vi "WLAN - TV - RW - UTIL - TestVectors_11B.vi"(0 "TV_IQComposite_11B":T2={"Standard"=0, "DSSS Demod Parameters"={"DSSS Auto Compute Acquisition Length Enabled"=0, "DSSS Equalization Enabled"=0, "DSSS Header Detection Enabled"=0, "DSSS MAC FCS Check Enabled"=0, "DSSS Measurement Start Location"=0, "DSSS Phase Tracking Method"=0, "DSSS Maximum Chips Used"=0, "DSSS Reference Pulse Shaping Filter"=0, "DSSS Reference Pulse Shaping Filter Coefficient"=0.0, "# Avg"=1024, "# Iterations"=1024, "DSSS Power Ramp Enabled"=0}, "DSSS Gen Paramaters"=[], "Measurement Enabled ? "=FALSE} {"DSSS Gen Paramaters"."Center Frequency(Hz)" format="%#_6p"; "DSSS Gen Paramaters"."Generation Properties"."DSSS Data Rate (Mbps)" items=["1", "2", "5.5 CCK", "5.5 PBCC", "11 CCK", "11 PBCC", "22", "33"]; "DSSS Demod Parameters"."DSSS Power Ramp Enabled" items=["False", "True"]; "DSSS Demod Parameters"."DSSS Auto Compute Acquisition Length Enabled" items=["False", "True"]; "DSSS Demod Parameters"."DSSS Phase Tracking Method" items=["Standard", "Instantaneous"]; "DSSS Demod Parameters"."DSSS Equalization Enabled" items=["False", "True"]; "DSSS Demod Parameters"."DSSS Reference Pulse Shaping Filter" items=["Rectangular", "Raised Cosine", "Root Raised Cosine", "Gaussian"]; "DSSS Demod Parameters"."DSSS MAC FCS Check Enabled" items=["False", "True"]; "DSSS Demod Parameters"."DSSS Header Detection Enabled" items=["False", "True"]; "Standard" items=["80211A/G/J/P OFDM", "80211B/G DSSS", "80211G DSSSOFDM", "80211N MIMOOFDM", "80211AC MIMOOFDM"]}, 1 "11b_Meas_Config":path, 3 "TV_802_11b":path, 9 "TV Paramaters":T1) -> ()   [LabVIEW 2011]
uses:
  Includes/WLAN - TV - RW - INC - TV_IQComposite_11B.ctl
  Includes/WLAN - TV - RW - INC - TV_DSSS Demod.ctl
  Includes/WLAN - TV - RW - INC - TV_Parameters.ctl
  Includes/WLAN - TV - RW - INC - Tx_Meas_Settings_DSSS_String.ctl
  <vilib>/Utility/file.llb/Write To Spreadsheet File (string).vi
panel:
  in  "Measurement Type 802.11G":enum32{"Tx Measurement", "Tx Measurement 2"}(tab)
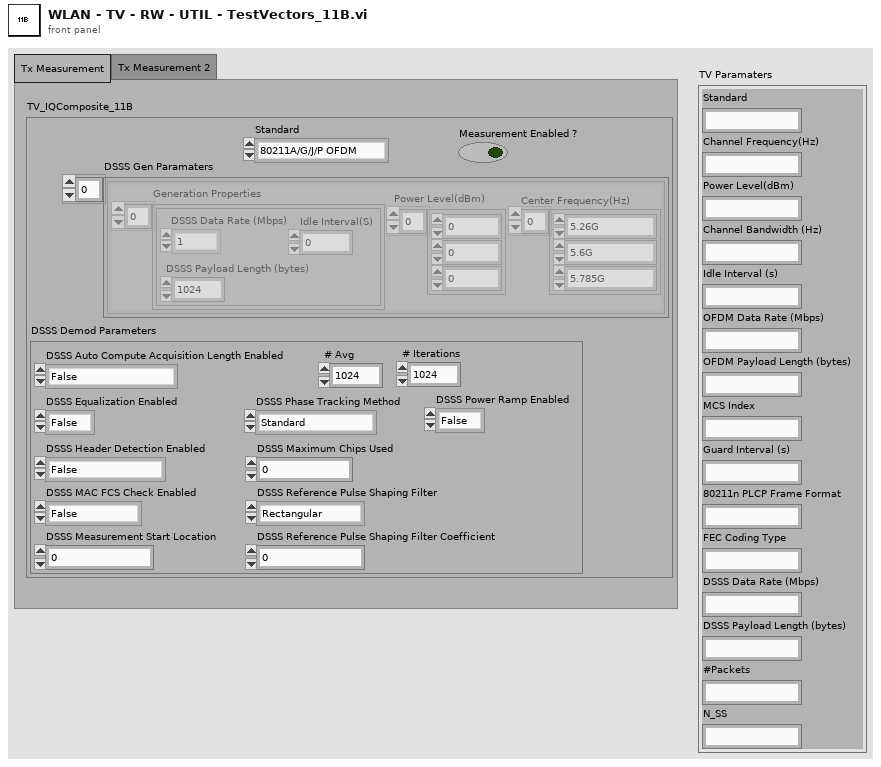
[diagram p1: front panel]
types:
  T1 = typedef "WLAN - TV - RW - INC - TV_Parameters.ctl" = cluster{"Standard ":string, "Channel Frequency(Hz)":string, "Power Level(dBm)":string, "Channel Bandwidth (Hz)":string, "Idle Interval (s)":string, "OFDM Data Rate (Mbps)":string, "OFDM Payload Length (bytes)":string, "MCS Index":string, "Guard Interval (s)":string, "80211n PLCP Frame Format":string, "FEC Coding Type":string, "DSSS Data Rate (Mbps)":string, "DSSS Payload Length (bytes)":string, "#Packets":string, "N_SS":string}
  T2 = typedef "WLAN - TV - RW - INC - TV_IQComposite_11B.ctl" = cluster{"Standard":i32, "DSSS Demod Parameters":T3, "DSSS Gen Paramaters":cluster{"Generation Properties":cluster{"DSSS Data Rate (Mbps)":i32, "DSSS Payload Length (bytes)":i32, "Idle Interval(S)":dbl}[], "Power Level(dBm)":dbl[], "Center Frequency(Hz)":dbl[]}[], "Measurement Enabled ? ":bool}
  T3 = typedef "WLAN - TV - RW - INC - TV_DSSS Demod.ctl" = cluster{"DSSS Auto Compute Acquisition Length Enabled":i32, "DSSS Equalization Enabled":i32, "DSSS Header Detection Enabled":i32, "DSSS MAC FCS Check Enabled":i32, "DSSS Measurement Start Location":i32, "DSSS Phase Tracking Method":i32, "DSSS Maximum Chips Used":i32, "DSSS Reference Pulse Shaping Filter":i32, "DSSS Reference Pulse Shaping Filter Coefficient":dbl, "# Avg":i32, "# Iterations":i32, "DSSS Power Ramp Enabled":i32}
  T4 = typedef "WLAN - TV - RW - INC - Tx_Meas_Settings_DSSS_String.ctl" = cluster{"DSSS Auto Compute Acquisition Length Enabled":string, "DSSS Equalization Enabled":string, "DSSS Header Detection Enabled":string, "DSSS MAC FCS Check Enabled":string, "DSSS Measurement Start Location":string, "DSSS Phase Tracking Method":string, "DSSS Maximum Chips Used":string, "DSSS Reference Pulse Shaping Filter":string, "DSSS Reference Pulse Shaping Filter Coefficient":string, "#Avg":string, "#Iterations":string, "DSSS Ramp Enabled ":string}
  T5 = cluster{"Generation Properties":cluster{"DSSS Data Rate (Mbps)":i32, "DSSS Payload Length (bytes)":i32, "Idle Interval(S)":dbl}[], "Power Level(dBm)":dbl[], "Center Frequency(Hz)":dbl[]}[]
  T6 = cluster{"DSSS Data Rate (Mbps)":i32, "DSSS Payload Length (bytes)":i32, "Idle Interval(S)":dbl}[]
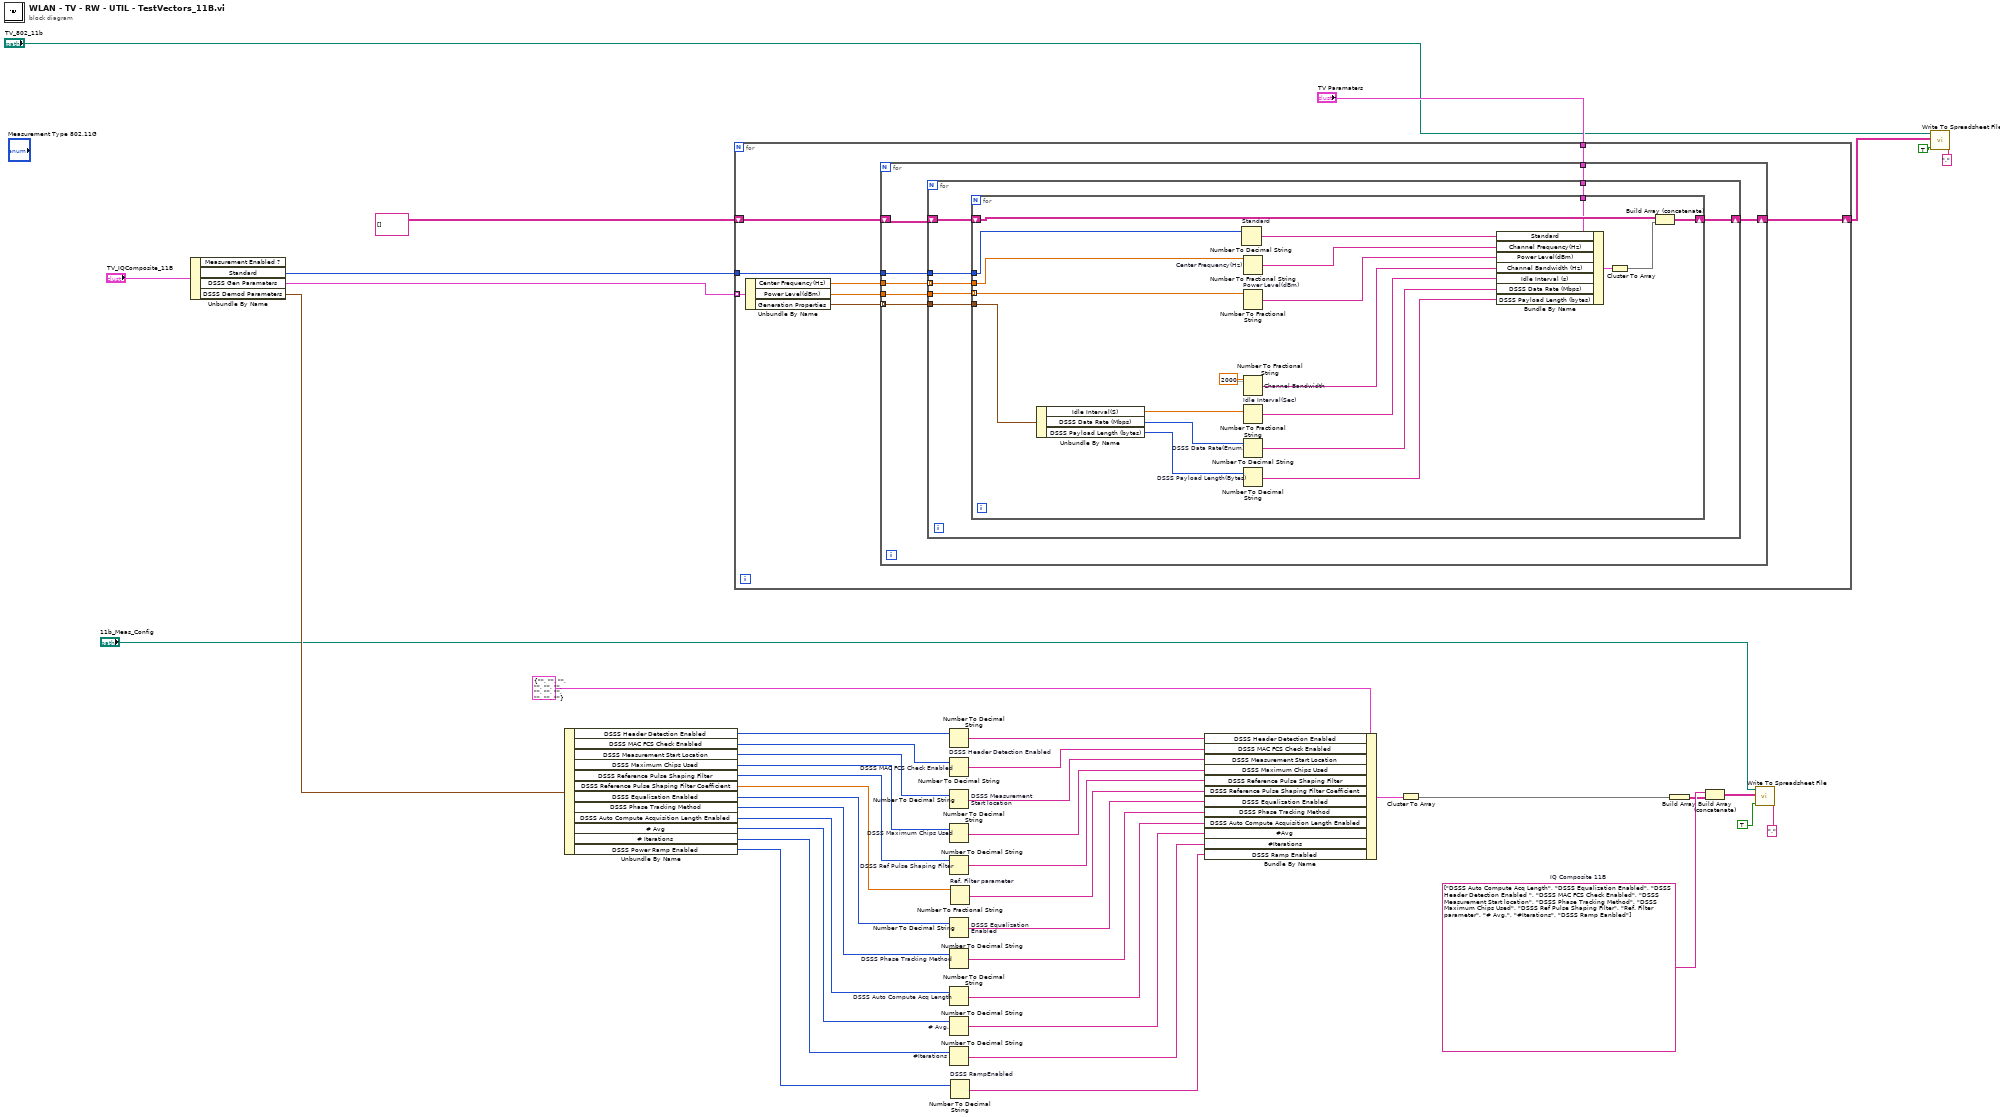
[diagram p0: block diagram]
diagram:
  w14 = string[] ["DSSS Auto Compute Acq Length", "DSSS Equalization Enabled", "DSSS Header Detection Enabled ", "DSSS MAC FCS Check Enabled", "DSSS Measurement Start location", "DSSS Phase Tracking Method", "DSSS Maximum Chips Used", "DSSS Ref Pulse Shaping Filter", "Ref. Filter parameter", "# Avg.", "#Iterations", "DSSS Ramp Eanbled"]  # IQ Composite 11B
  n1 = Unbundle By Name("TV_IQComposite_11B") -> ("Standard"=w40:i32, "DSSS Gen Paramaters"=w43:T5, "DSSS Demod Parameters"=w11:T3)  [unwired: 1 out]
  n2 = Unbundle By Name(w11) -> ("DSSS Header Detection Enabled"=w27:i32, "DSSS MAC FCS Check Enabled"=w28:i32, "DSSS Measurement Start Location"=w29:i32, "DSSS Maximum Chips Used"=w30:i32, "DSSS Reference Pulse Shaping Filter"=w31:i32, "DSSS Reference Pulse Shaping Filter Coefficient"=w7:dbl, "DSSS Equalization Enabled"=w32:i32, "DSSS Phase Tracking Method"=w33:i32, "DSSS Auto Compute Acquisition Length Enabled"=w34:i32, "# Avg"=w35:i32, "# Iterations"=w36:i32, "DSSS Power Ramp Enabled"=w6:i32)
  n3 = for {
    tunnel: w43 -> [w48] mode=indexing
    tunnel: w40 -> [w51]
    tunnel: "TV Paramaters" -> [w49]
    shift-right: [w50] -> w1
    shift-left: string[][] [] ("appended array") -> [w44]
    n4 = Unbundle By Name(w48) -> ("Center Frequency(Hz)"=w47:dbl[], "Power Level(dBm)"=w46:dbl[], "Generation Properties"=w45:T6)
    n5 = for {
      tunnel: w47 -> [w58]
      tunnel: w46 -> [w57]
      tunnel: w45 -> [w56] mode=indexing
      tunnel: w51 -> [w55]
      tunnel: w49 -> [w53]
      shift-right: [w54] -> w50
      shift-left: w44 -> [w52]
      n6 = for {
        tunnel: w58 -> [w63] mode=indexing
        tunnel: w57 -> [w65]
        tunnel: w56 -> [w64]
        shift-right: [w61] -> w54
        shift-left: w52 -> [w62]
        tunnel: w55 -> [w60]
        tunnel: w53 -> [w59]
        n7 = for {
          tunnel: w65 -> [w68] mode=indexing
          tunnel: w64 -> [w72]
          tunnel: w63 -> [w69]
          shift-right: [w85] -> w61
          shift-left: w62 -> [w84]
          tunnel: w60 -> [w83]
          tunnel: w59 -> [w81]
          n8 = Unbundle By Name(w72) -> ("Idle Interval(S)"=w70:dbl, "DSSS Data Rate (Mbps)"=w73:i32, "DSSS Payload Length (bytes)"=w71:i32)
          n9 = Number To Decimal String "Standard"(number=w83) -> (decimal integer string=w74:string)  [unwired: 1 in]
          n10 = Number To Fractional String "Center Frequency(Hz)"(number=w69) -> (F-format string=w75:string)  [unwired: 3 in]
          n11 = Number To Fractional String "Power Level(dBm)"(number=w68) -> (F-format string=w76:string)  [unwired: 3 in]
          n12 = Number To Fractional String "Channel Bandwidth"(number=20000000.0) -> (F-format string=w77:string)  [unwired: 3 in]
          n13 = Number To Fractional String "Idle Interval(Sec)"(number=w70) -> (F-format string=w78:string)  [unwired: 3 in]
          n14 = Number To Decimal String "DSSS Data Rate(Enum)"(number=w73) -> (decimal integer string=w79:string)  [unwired: 1 in]
          n15 = Number To Decimal String "DSSS Payload Length(Bytes)"(number=w71) -> (decimal integer string=w80:string)  [unwired: 1 in]
          n16 = Bundle By Name(cluster=w81, "Standard"=w74, "Channel Frequency(Hz)"=w75, "Power Level(dBm)"=w76, "Channel Bandwidth (Hz)"=w77, "Idle Interval (s)"=w78, "DSSS Data Rate (Mbps)"=w79, "DSSS Payload Length (bytes)"=w80) -> (w67:T1)
          n17 = Cluster To Array(cluster=w67) -> (array=w66:string[])
          n18 = Build Array (concatenate)(w84, w66) -> (w85:string[][])
        }
      }
    }
  }
  n19 = Number To Decimal String "DSSS Header Detection Enabled"(number=w27) -> (decimal integer string=w26:string)  [unwired: 1 in]
  n20 = Number To Decimal String "DSSS MAC FCS Check Enabled"(number=w28) -> (decimal integer string=w25:string)  [unwired: 1 in]
  n21 = Number To Decimal String "DSSS Measurement Start location"(number=w29) -> (decimal integer string=w24:string)  [unwired: 1 in]
  n22 = Number To Decimal String "DSSS Maximum Chips Used"(number=w30) -> (decimal integer string=w23:string)  [unwired: 1 in]
  n23 = Number To Decimal String "DSSS Ref Pulse Shaping Filter"(number=w31) -> (decimal integer string=w22:string)  [unwired: 1 in]
  n24 = Number To Decimal String "DSSS Equalization Enabled"(number=w32) -> (decimal integer string=w17:string)  [unwired: 1 in]
  n25 = Number To Decimal String "DSSS Phase Tracking Method"(number=w33) -> (decimal integer string=w18:string)  [unwired: 1 in]
  n26 = Number To Decimal String "DSSS Auto Compute Acq Length"(number=w34) -> (decimal integer string=w19:string)  [unwired: 1 in]
  n27 = Number To Decimal String "# Avg."(number=w35) -> (decimal integer string=w20:string)  [unwired: 1 in]
  n28 = Number To Decimal String "#Iterations"(number=w36) -> (decimal integer string=w21:string)  [unwired: 1 in]
  n29 = Number To Decimal String "DSSS RampEnabled"(number=w6) -> (decimal integer string=w5:string)  [unwired: 1 in]
  n30 = Number To Fractional String "Ref. Filter parameter"(number=w7) -> (F-format string=w8:string)  [unwired: 3 in]
  n31 = Bundle By Name(cluster=T4 {"DSSS Auto Compute Acquisition Length Enabled"="", "DSSS Equalization Enabled"="", "DSSS Header Detection Enabled"="", "DSSS MAC FCS Check Enabled"="", "DSSS Measurement Start Location"="", "DSSS Phase Tracking Method"="", "DSSS Maximum Chips Used"="", "DSSS Reference Pulse Shaping Filter"="", "DSSS Reference Pulse Shaping Filter Coefficient"="", "#Avg"="", "#Iterations"="", "DSSS Ramp Enabled "=""} ("OFDM Measurement Settings"), "DSSS Header Detection Enabled"=w26, "DSSS MAC FCS Check Enabled"=w25, "DSSS Measurement Start Location"=w24, "DSSS Maximum Chips Used"=w23, "DSSS Reference Pulse Shaping Filter"=w22, "DSSS Reference Pulse Shaping Filter Coefficient"=w8, "DSSS Equalization Enabled"=w17, "DSSS Phase Tracking Method"=w18, "DSSS Auto Compute Acquisition Length Enabled"=w19, "#Avg"=w20, "#Iterations"=w21, "DSSS Ramp Enabled"=w5) -> (w4:T4)
  n32 = Cluster To Array(cluster=w4) -> (array=w3:string[])
  n33 = Build Array(w3) -> (w12:string[][])
  n34 = Build Array (concatenate)(w14, w12) -> (w13:string[][])
  n35 = call-poly <vilib>:"Write To Spreadsheet File.vi"("delimiter (\\t)"="," ("delimiter (\\t)"), "append to file? (new file:F)"=TRUE, "2D data"=w13, "file path (dialog if empty)"="11b_Meas_Config") -> ()  [unwired: 4 in, 1 out]
  n36 = call-poly <vilib>:"Write To Spreadsheet File.vi"("delimiter (\\t)"="," ("delimiter (\\t)"), "append to file? (new file:F)"=TRUE, "2D data"=w1, "file path (dialog if empty)"="TV_802_11b") -> ()  [unwired: 4 in, 1 out]
